vi "配置说明.vi"() -> (3 "字符串":string)   [LabVIEW 2016, in "环境动力监测库.lvlib"]
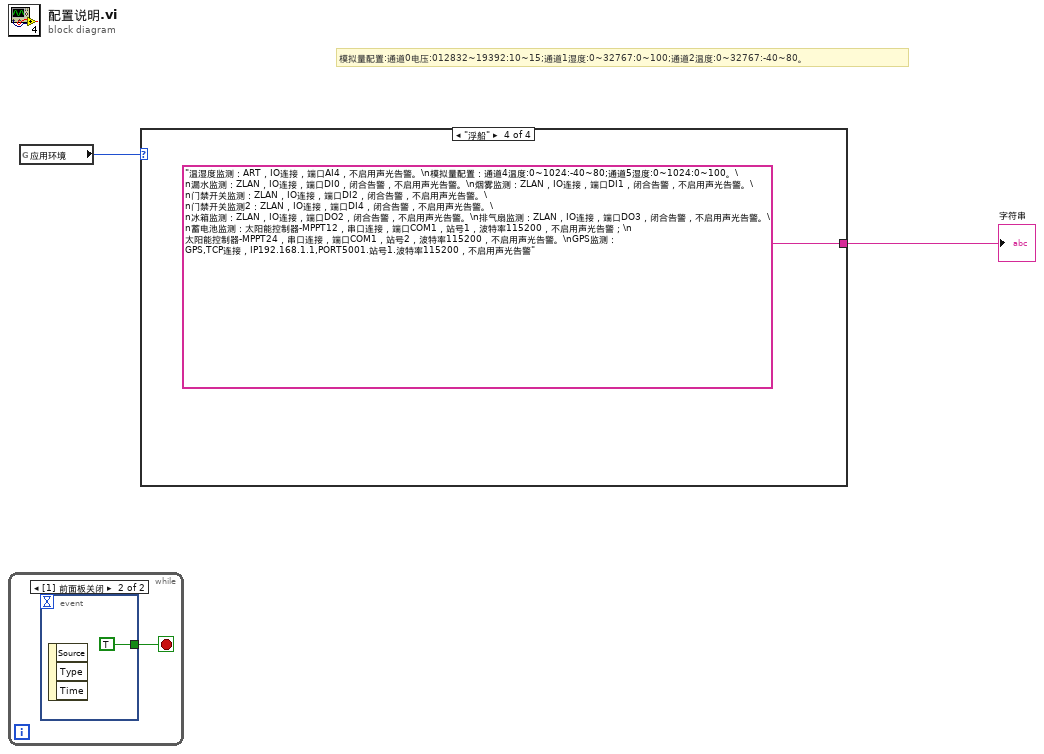
[diagram p0: block diagram]
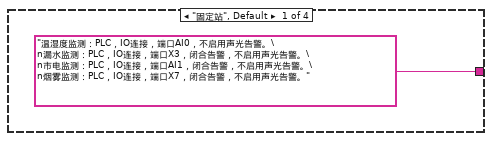
[diagram p2: hidden frame]
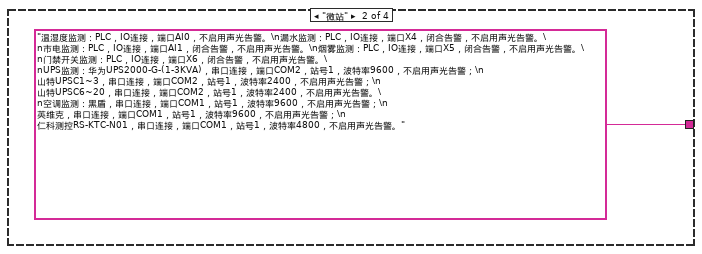
[diagram p3: hidden frame]
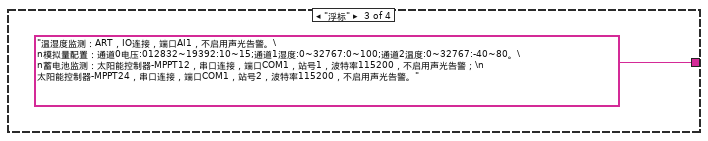
[diagram p4: hidden frame]
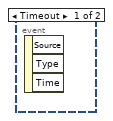
[diagram p5: hidden frame]
diagram:
  # "模拟量配置:通道0电压:012832~19392:10~15;通道1湿度:0~32767:0~100;通道2温度:0~32767:-40~80。"
  n1 = while {
    stop <- w3 stop-if-true
    n2 = event shown="[1] 前面板关闭" {
      selector: _ -> [_ _]
      dyn-events: _ -> [_ _]
      timeout: _ -> [_ _]
      tunnel: [_ TRUE] -> w3
      event Timeout {
        n3 = event-data() -> ()  [unwired: 1 in, 3 out]
      }
      event Panel Close {
        n4 = event-data() -> ()  [unwired: 1 in, 3 out]
      }
    }
  }
  n5 = global read "外部交互全局变量.vi" "应用环境"() -> (w1:enum16{"固定站", "微站", "浮标", "浮船"})
  n6 = case shown="\"浮船\"" w1 {
    tunnel: ["温湿度监测：PLC，IO连接，端口AI0，不启用声光告警。\n漏水监测：PLC，IO连接，端口X3，闭合告警，不启用声光告警。\n市电监测：PLC，IO连接，端口AI1，闭合告警，不启用声光告警。\n烟雾监测：PLC，IO连接，端口X7，闭合告警，不启用声光告警。" ("字符串") "温湿度监测：PLC，IO连接，端口AI0，不启用声光告警。\n漏水监测：PLC，IO连接，端口X4，闭合告警，不启用声光告警。\n市电监测：PLC，IO连接，端口AI1，闭合告警，不启用声光告警。\n烟雾监测：PLC，IO连接，端口X5，闭合告警，不启用声光告警。\n门禁开关监测：PLC，IO连接，端口X6，闭合告警，不启用声光告警。\nUPS监测：华为UPS2000-G-(1-3KVA)，串口连接，端口COM2，站号1，波特率9600，不启用声光告警；\n                  山特UPSC1~3，串口连接，端口COM2，站号1，波特率2400，不启用声光告警；\n                  山特UPSC6~20，串口连接，端口COM2，站号1，波特率2400，不启用声光告警。\n空调监测：黑盾，串口连接，端口COM1，站号1，波特率9600，不启用声光告警；\n                  英维克，串口连接，端口COM1，站号1，波特率9600，不启用声光告警；\n                  仁科测控RS-KTC-N01，串口连接，端口COM1，站号1，波特率4800，不启用声光告警。" ("字符串") "温湿度监测：ART，IO连接，端口AI1，不启用声光告警。\n模拟量配置：通道0电压:012832~19392:10~15;通道1湿度:0~32767:0~100;通道2温度:0~32767:-40~80。\n蓄电池监测：太阳能控制器-MPPT12，串口连接，端口COM1，站号1，波特率115200，不启用声光告警；\n                  太阳能控制器-MPPT24，串口连接，端口COM1，站号2，波特率115200，不启用声光告警。" ("字符串") "温湿度监测：ART，IO连接，端口AI4，不启用声光告警。\n模拟量配置：通道4温度:0~1024:-40~80;通道5湿度:0~1024:0~100。\n漏水监测：ZLAN，IO连接，端口DI0，闭合告警，不启用声光告警。\n烟雾监测：ZLAN，IO连接，端口DI1，闭合告警，不启用声光告警。\n门禁开关监测：ZLAN，IO连接，端口DI2，闭合告警，不启用声光告警。\n门禁开关监测2：ZLAN，IO连接，端口DI4，闭合告警，不启用声光告警。\n冰箱监测：ZLAN，IO连接，端口DO2，闭合告警，不启用声光告警。\n排气扇监测：ZLAN，IO连接，端口DO3，闭合告警，不启用声光告警。\n蓄电池监测：太阳能控制器-MPPT12，串口连接，端口COM1，站号1，波特率115200，不启用声光告警；\n                     太阳能控制器-MPPT24，串口连接，端口COM1，站号2，波特率115200，不启用声光告警。\nGPS监测： GPS,TCP连接，IP192.168.1.1,PORT5001.站号1.波特率115200，不启用声光告警" ("字符串")] -> w2
    frame "固定站", Default {
    }
    frame "微站" {
    }
    frame "浮标" {
    }
    frame "浮船" {
    }
  }
  "字符串" <- w2
